vi "GetPayloadDVR.vi"(7 "Msg":refnum<class "Msg.lvclass">) -> (3 "PayloadDVR":refnum<data-value>)   [LabVIEW 2020, in "_Template.lvlib" / "{{Msg}}.lvlib" / "Msg.lvclass"]
uses:
  Msg.lvclass
  Payload.ctl
  Msg.lvclass/Msg.ctl
  {{Msg}}.lvlib
panel:
  # "This front panel should not be manipulated."
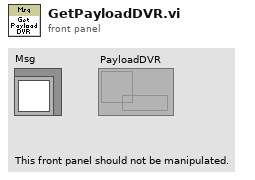
[diagram p1: front panel]
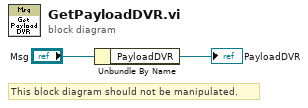
[diagram p0: block diagram]
diagram:
  # "This block diagram should not be manipulated."
  n1 = Unbundle By Name("Msg") -> ("PayloadDVR"=→"PayloadDVR":refnum<data-value>)
